vi "cs_usb_write.vi"(3 "string to send":string, 4 "btc_pipe":i32=1, 5 "handle":i32=272) -> (0 "Error":bool)   [LabVIEW 2017]
uses:
  kernel32.dll
panel:
  in  "Case Constant\n(See Context Help)":bool
  out "bufOutput":u8[](array[numeric])=[103, 111, 119, 97, 118, 101, 32, 48, 13, 10] format="%x"
  out "size 2":i32
  in  "btc_byteArray":u8[](array[numeric])
  in  "BULK_TRANSFER_CONTROL":cluster{"Numeric":u32}={"Numeric"=1}
  in  "overlapp":i32
  in  "size":i32
  out "outp-size":i32=64
  out "btc-size":i32=3
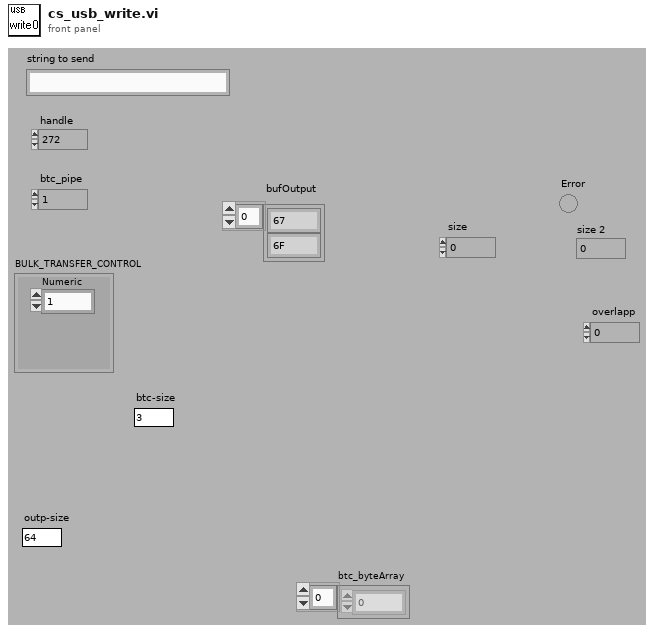
[diagram p1: front panel]
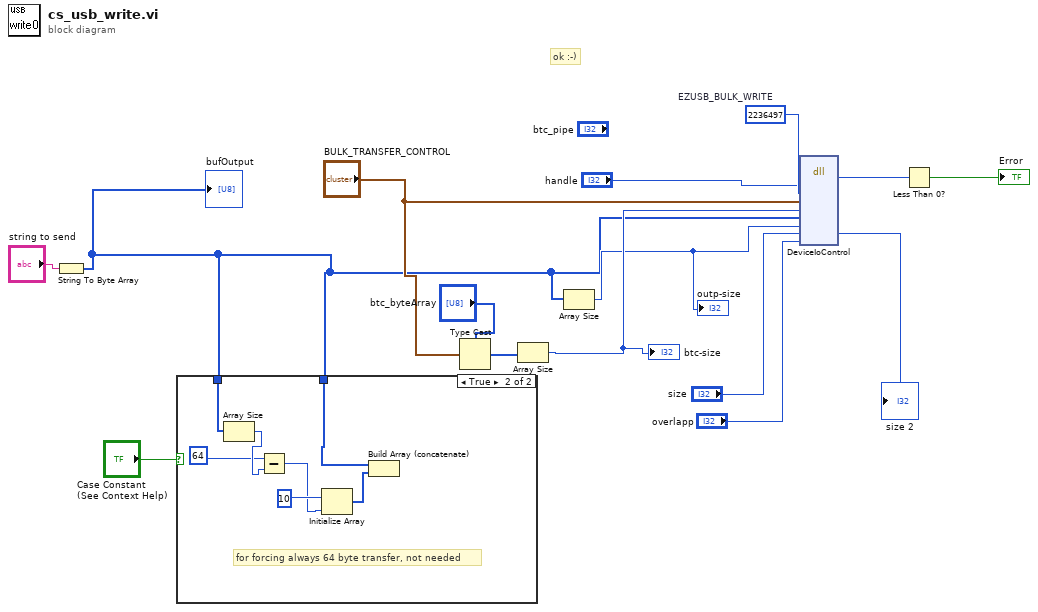
[diagram p0: block diagram]
diagram:
  w15 = u32 2236497  # EZUSB_BULK_WRITE
  # "ok :-)"
  n1 = String To Byte Array(string="string to send") -> (unsigned byte array=w1:u8[])
  "bufOutput" <- w1
  n2 = case shown="True" "Case Constant\n(See Context Help)" {
    tunnel: w1 -> [_ w18]
    tunnel: w1 -> [_ w16]
    frame False {
    }
    frame True {
      # "for forcing always 64 byte transfer, not needed"
      n3 = Array Size(array=w16) -> (size(s)=w21:i32)
      n4 = Subtract(x=u8 64, y=w21) -> (x-y=w20:i32)
      n5 = Initialize Array(u8 10, w20) -> (w19:u8[])
      n6 = Build Array (concatenate)(w18, w19) -> ()  [unwired: 1 out]
    }
  }
  n7 = Type Cast(type="btc_byteArray", x="BULK_TRANSFER_CONTROL") -> (*(type *) &x=w8:u8[])
  n8 = Array Size(array=w8) -> (size(s)=w7:i32)
  "btc-size" <- w7
  n9 = Array Size(array=w1) -> (size(s)=w4:i32)
  "outp-size" <- w4
  n10 = dll-call lib="kernel32.dll" fn="DeviceIoControl" label="DeviceIOControl"("handle"="handle", "vier-const"=w15, "BULK_TRANSFER_CONTROL"="BULK_TRANSFER_CONTROL", "inputsize"=w7, "output"=w1, "outputsize"=w4, "size"="size", "overlapp"="overlapp") -> ("ltemp"=w10:i32, "size"=→"size 2":i32)  [unwired: 10 in, 2 out]
  n11 = Less Than 0?(x=w10) -> (x < 0?=→"Error":bool)
